vi "Select and Run Tests on Disk.vi"(4 "Verbose":bool=TRUE, 5 "Silent":bool, 6 "Interactive":bool=TRUE, 7 "Inspect Recursively":bool=TRUE, 9 "Report name":string, 10 "Output Folder":path, 11 "Source Folder":path) -> ()   [LabVIEW 2013]
uses:
  subVIs/Run Tests Programmatically.vi
  Caraya.lvlib
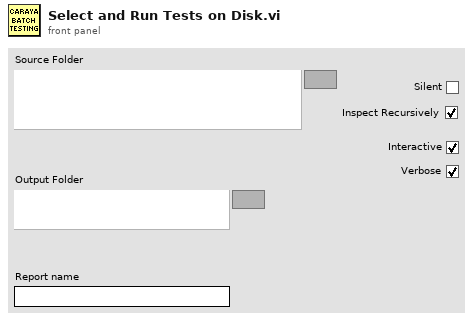
[diagram p1: front panel]
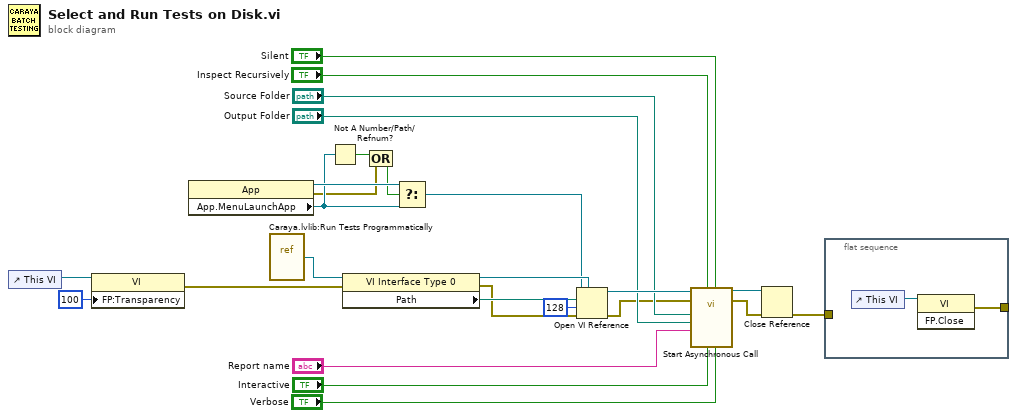
[diagram p0: block diagram]
diagram:
  n1 = control-ref of="This VI"() -> (w9:refnum<vi>)
  n2 = property class="VI"(reference=w9, "FP:Transparency"=u8 100 ("Front Panel Window:Transparency")) -> (error out=w7:errorcluster)  [unwired: 1 in, 1 out]
  n3 = property class="App"() -> (reference out=w6:refnum<vi>, error out=w4:errorcluster, "App.MenuLaunchApp"=w5:refnum<vi>)  [unwired: 2 in]
  n4 = vi-ref "Caraya.lvlib:Run Tests Programmatically.vi"() -> (w16:refnum<vi>)
  n5 = Not A Number/Path/Refnum?(number/path/refnum=w5) -> (NaN/Path/Refnum?=w3:bool)
  n6 = property class="VI Interface Type 0"(reference=w16, error in=w7) -> (reference out=w15:refnum<vi>, error out=w13:errorcluster, "Path"=w17:path)
  n7 = Compound Arithmetic op=OR(w3, w4) -> (w2:bool)
  n8 = Select(t=w6, s=w2, f=w5) -> (s? t:f=w1:refnum<vi>)
  n9 = Open VI Reference(type specifier VI Refnum (for type only)=w15, application reference (local)=w1, vi path=w17, options=128, error in (no error)=w13) -> (vi reference=w26:refnum<vi>, error out=w14:errorcluster)  [unwired: 1 in]
  n10 = call-by-ref "Start Asynchronous Call"(reference=w26, error in=w14, "Verbose"="Verbose", "Silent"="Silent", "Interactive"="Interactive", "Inspect Recursively"="Inspect Recursively", "Report name"="Report name", "Output Folder"="Output Folder", "Source Folder"="Source Folder") -> (reference out=w12:refnum<vi>, error out=w11:errorcluster)  [unwired: 3 in, 2 out]
  n11 = Close Reference(reference=w12, error in (no error)=w11) -> (error out=w10:errorcluster)
  n12 = flat-sequence {
    tunnel: w10 -> [_]
    tunnel: [w27] -> _
    frame #0 {
      n13 = control-ref of="This VI"() -> (w28:refnum<vi>)
      n14 = invoke class="VI" method="FP.Close"(reference=w28) -> (error out=w27:errorcluster)  [unwired: 2 in, 2 out]
    }
  }
